vi "Player Info.vi"(11 "64 in":refnum<class "Picture.lvclass">) -> (0 "Defeat Speech":string, 1 "Victory Speech":string, 2 "Name":string, 3 "64 out":refnum<class "Picture.lvclass">)   [LabVIEW 2020, in "Picture.lvclass"]
uses:
  Picture.lvclass
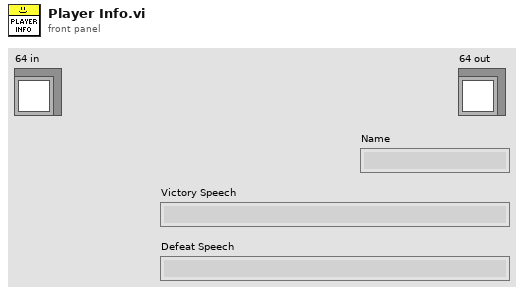
[diagram p1: front panel]
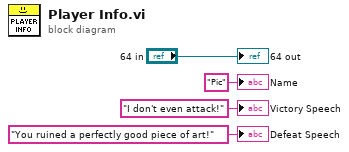
[diagram p0: block diagram]
diagram:
  "64 out" <- "64 in"
  "Name" <- "Pic" ("Name")
  "Victory Speech" <- "I don't even attack!" ("Victory Speech")
  "Defeat Speech" <- "You ruined a perfectly good piece of art!" ("Defeat Speech")
